vi "Mod_OFDM_Add_Cylic_Prefix_Frame.vi"(0 "Complex IFFT":cdb[][](array[numeric]), 7 "Parameters per Ofdm Symbol":T1 {"Data Source"."Data Source"."Register Initial State" format="%08x"}, 11 "error in":errorcluster) -> (4 "Complex Symbols w/  Cyclic prefix":cdb[](array[numeric]), 6 "Complex IFFT w/ Cyclic Prefix":cdb[][](array[numeric]), 15 "error out":errorcluster)   [LabVIEW 2010]
doc: "After performing an IFFT, the output is cyclically extended to the desired length by prepending the output of the IFFT."
uses:
  Controls(Type_DEf)/Parameters per Ofdm Symbol.ctl
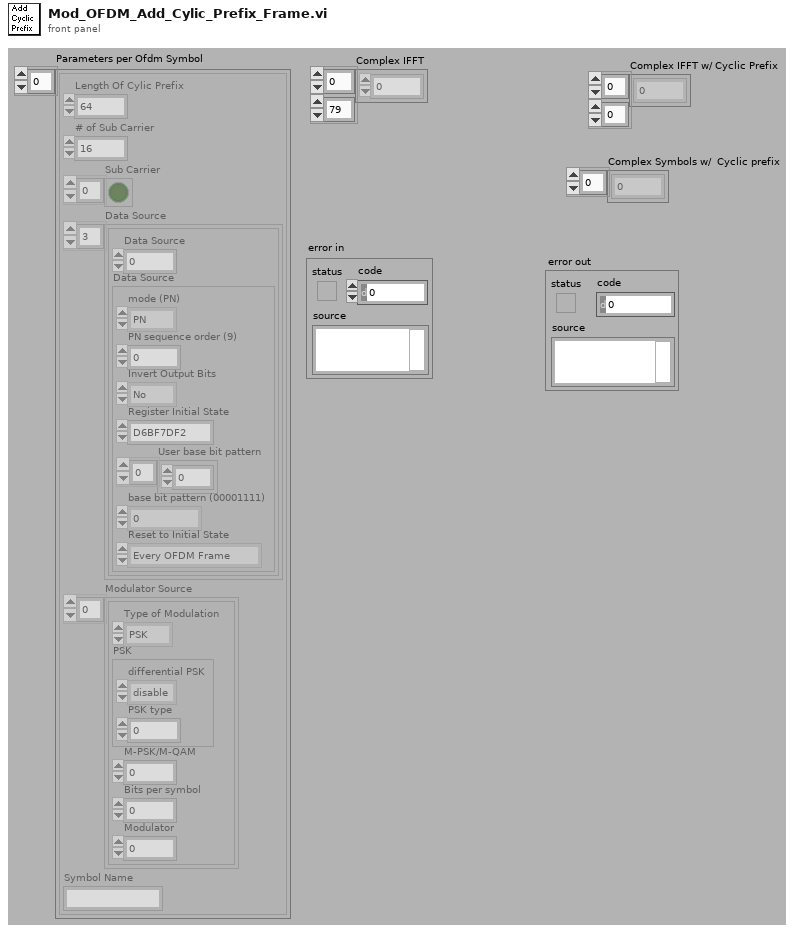
[diagram p1: front panel]
types:
  T1 = typedef "Parameters per Ofdm Symbol.ctl" = cluster{"Length Of Cylic Prefix":i32, "# of Sub Carrier":i32, "Sub Carrier":bool[], "Data Source":cluster{"Data Source":u16, "Data Source":cluster{"mode (PN)":enum16{"PN", "pattern", "user"}, "PN sequence order (9)":i32, "Invert Output Bits":enum16{"No", "Yes"}, "Register Initial State":u32, "User base bit pattern":i8[], "base bit pattern (00001111)":enum16{"0", "1", "01", "0011", "00001111"}, "Reset to Initial State":enum16{"Every OFDM Frame", "Every OFDM Symbol", "Every Sub Carrier"}}}[], "Modulator Source":cluster{"Type of Modulation":enum16{"PSK", "QAM"}, "PSK":cluster{"differential PSK":enum16{"disable", "enable"}, "PSK type":u16}, "M-PSK/M-QAM":i32, "Bits per symbol":i32, "Modulator":u16}[], "Symbol Name":string}[]
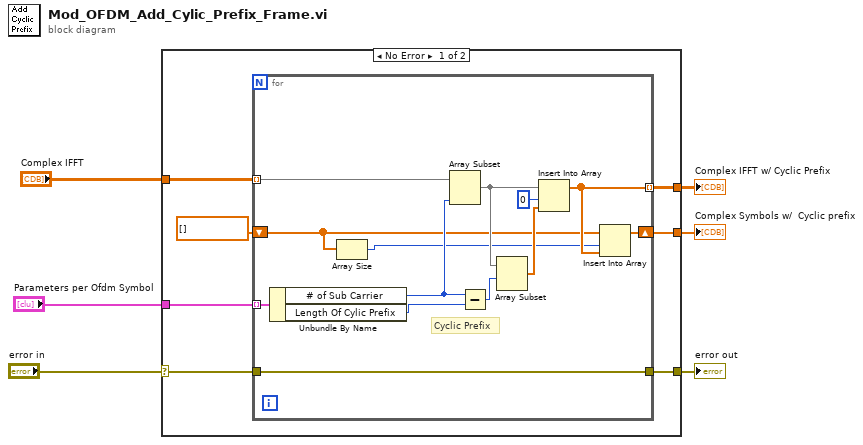
[diagram p0: block diagram]
diagram:
  n1 = case shown="No Error" "error in" {
    selector: "error in" -> [w7 w27]
    tunnel: "Complex IFFT" -> [w13 _]
    tunnel: "Parameters per Ofdm Symbol" -> [w12 _]
    tunnel: [w11 _] -> w4
    tunnel: [w10 w27] -> w3
    tunnel: [w8 _] -> w2
    frame No Error {
      n2 = for {
        tunnel: w13 -> [w21] mode=indexing
        tunnel: w12 -> [w20] mode=indexing
        tunnel: [w16] -> w11 mode=indexing
        tunnel: w7 -> [w18]
        tunnel: [w18] -> w10
        shift-right: [w17] -> w8
        shift-left: cdb[] [] -> [w15]
        # "Cyclic Prefix"
        n3 = Unbundle By Name(w20) -> ("# of Sub Carrier"=w25:i32, "Length Of Cylic Prefix"=w19:i32)
        n4 = Array Size(array=w15) -> (size(s)=w14:i32)
        n5 = Array Subset(array=w21, length=w25) -> (w24:cdb[])  [unwired: 1 in]
        n6 = Subtract(x=w25, y=w19) -> (x-y=w26:i32)
        n7 = Array Subset(array=w24, index=w26) -> (w23:cdb[])  [unwired: 1 in]
        n8 = Insert Into Array(array=w24, index=0, new element=w23) -> (w16:cdb[])
        n9 = Insert Into Array(array=w15, index=w14, new element=w16) -> (w17:cdb[])
      }
    }
    frame Error {
    }
  }
  "Complex IFFT w/ Cyclic Prefix" <- w4
  "error out" <- w3
  "Complex Symbols w/  Cyclic prefix" <- w2
